vi "AB_Engine_AddVisitedVI.vi"(9 "New Item":T1, 10 "Visited VIs Hash":variant, 11 "Visited VIs Array":T1[](array[typedef])) -> (2 "Visited VIs Hash":variant, 3 "Visited VIs Array out":T1[](array[typedef]))   [LabVIEW 2020]
uses:
  <vilib>/AppBuilder/Engine/AB_Engine_PathNode.ctl
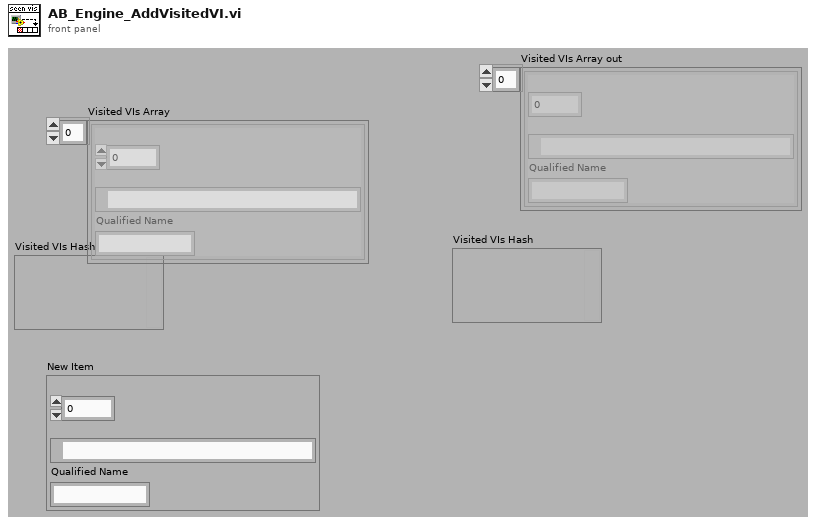
[diagram p1: front panel]
types:
  T1 = typedef "AB_Engine_PathNode.ctl" = cluster{"parent":i32, "path":path, "Qualified Name":string}
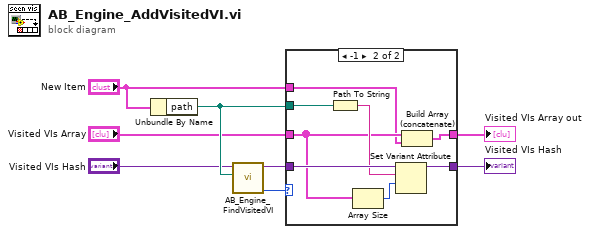
[diagram p0: block diagram]
diagram:
  n1 = Unbundle By Name("New Item") -> ("path"=w8:path)
  n2 = call <vilib>:"AB_Engine_FindVisitedVI.vi"("path"=w8, "hash table"="Visited VIs Hash") -> ("index of element"=w2:i32, "hash table out"=w6:variant)  [unwired: 7 in, 1 out]
  n3 = case shown="-1" w2 {
    tunnel: [w10 w18] -> w1
    tunnel: "Visited VIs Array" -> [w10 w14]
    tunnel: w6 -> [w9 w17]
    tunnel: [w9 w13] -> w5
    tunnel: "New Item" -> [_ w12]
    tunnel: w8 -> [_ w11]
    frame 0, Default {
    }
    frame -1 {
      n4 = Path To String(path=w11) -> (string=w16:string)
      n5 = Array Size(array=w14) -> (size(s)=w15:i32)
      n6 = Set Variant Attribute(Variant=w17, name=w16, value=w15) -> (Variant out=w13:variant)  [unwired: 1 in, 2 out]
      n7 = Build Array (concatenate)(w14, w12) -> (w18:T1[])
    }
  }
  "Visited VIs Hash" <- w5
  "Visited VIs Array out" <- w1
